vi "短信通知-发送.vi"(11 "探头名称":string) -> ()   [LabVIEW 2017]
uses:
  <vilib>/httpClient/LabVIEWHTTPClient.lvlib
panel:
  out "headers":string caption="头部"
  out "body":string caption="体部"
  out "短信内容":string
  out "Result":string caption="结果"
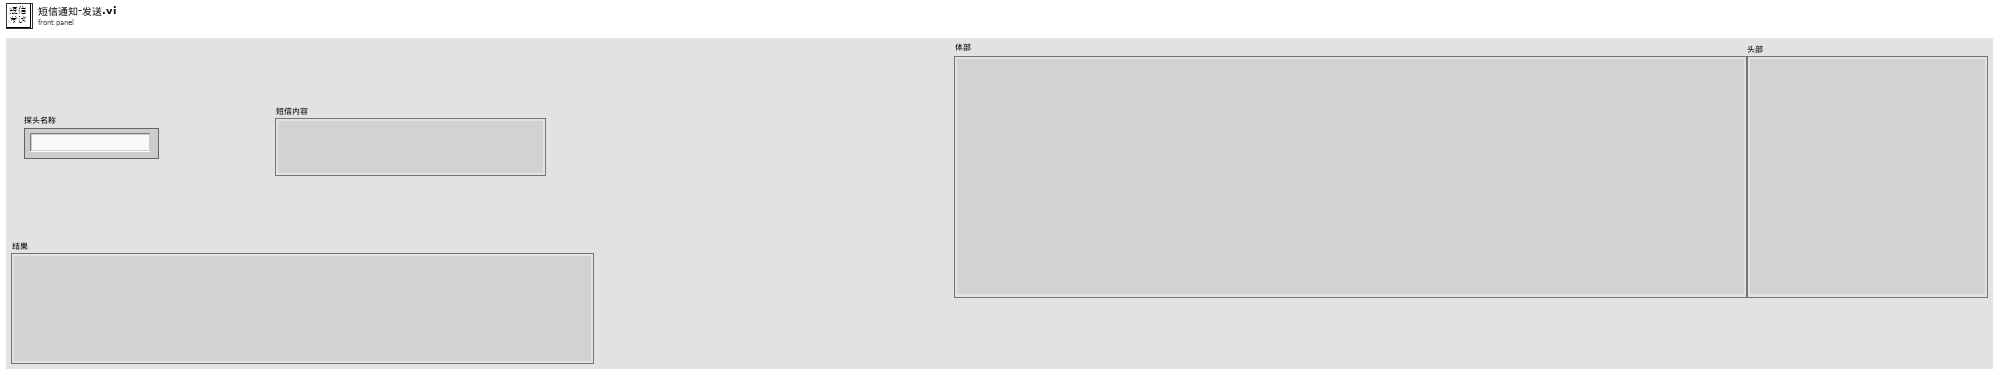
[diagram p1: front panel]
types:
  T1 = cluster{"企业编号":string, "员工编号":string, "通道号":string, "密码":string, "联系人数组":cluster{"姓名":string, "手机号":string}[]}
  T2 = typedef "LabVIEWHTTPClient.lvlib/ClientHandle.ctl" = refnum<k1>
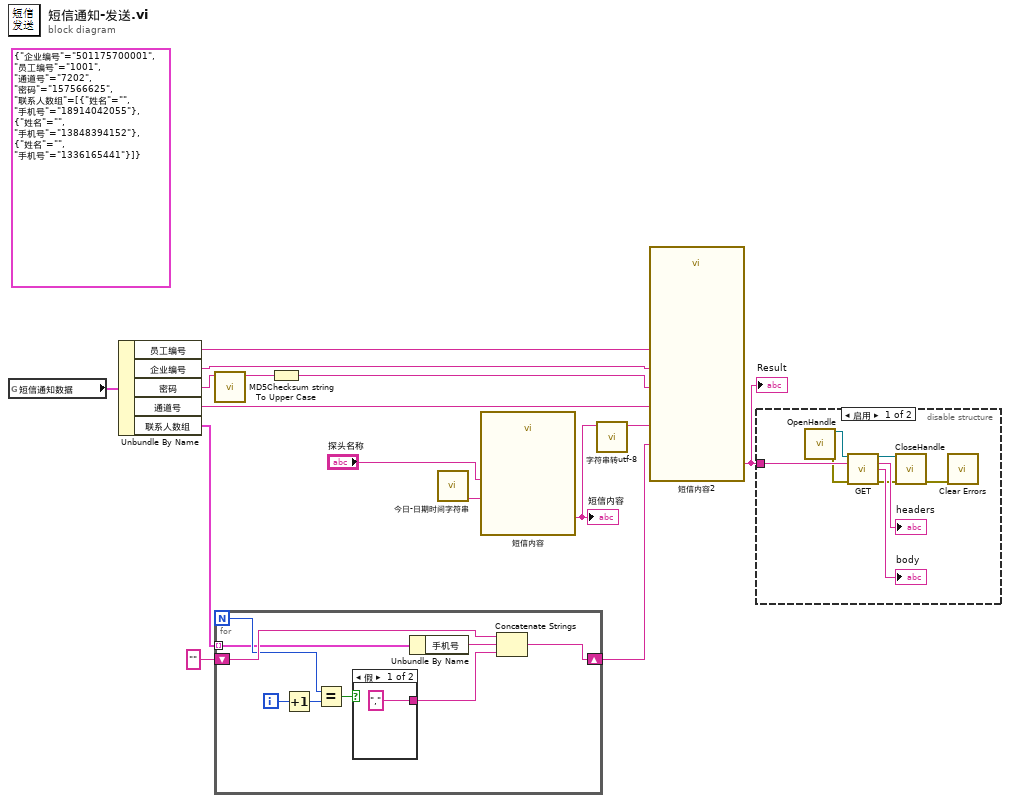
[diagram p0: block diagram]
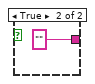
[diagram p3: hidden frame]
diagram:
  (unwired) T1 {"企业编号"="501175700001", "员工编号"="1001", "通道号"="7202", "密码"="157566625", "联系人数组"=[{"姓名"="", "手机号"="18914042055"}, {"姓名"="", "手机号"="13848394152"}, {"姓名"="", "手机号"="1336165441"}]} ("短信通知数据")
  n1 = global read "全局变量-35点监测.vi" "短信通知数据"() -> (w1:T1)
  n2 = Unbundle By Name(w1) -> ("员工编号"=w15:string, "企业编号"=w14:string, "密码"=w12:string, "通道号"=w13:string, "联系人数组"=w9:cluster{"姓名":string, "手机号":string}[])
  n3 = call <vilib>:"MD5Checksum string.vi"("Message String"=w12) -> ("MD5 message-digest"=w11:string)  [unwired: 10 in]
  n4 = for {
    N -> [w19]
    tunnel: w9 -> [w17] mode=indexing
    shift-right: [w23] -> w7
    shift-left: "" -> [w24]
    i -> [w21]
    n5 = Increment(x=w21) -> (x+1=w20:i32)
    n6 = Equal?(x=w19, y=w20) -> (x = y?=w18:bool)
    n7 = case shown="假" w18 {
      tunnel: ["," ("字符串") "" ("字符串")] -> w22
      frame False {
      }
      frame True {
      }
    }
    n8 = Unbundle By Name(w17) -> ("手机号"=w16:string)
    n9 = Concatenate Strings(w24, w16, w22) -> (w23:string)
  }
  n10 = To Upper Case(1:w11) -> (0:w10:string)
  n11 = call "今日-日期时间字符串.vi"() -> ("日期时间"=w4:string)  [unwired: 9 in, 2 out]
  n12 = call "短信内容"("探头名称"="探头名称", "时间"=w4) -> ("Result"=w3:string)  [unwired: 12 in, 1 out]
  "短信内容" <- w3
  n13 = call "字符串转utf-8.vi"("文本"=w3) -> ("utf-8文本"=w6:string)  [unwired: 9 in, 1 out]
  n14 = call "短信内容2"("通道号"=w13, "手机号s"=w7, "员工编号"=w15, "企业编号"=w14, "MD5密码"=w10, "短信内容"=w6) -> ("Result"=w2:string)  [unwired: 8 in, 1 out]
  "Result" <- w2
  n15 = disable-structure shown="启用" {
    disable-tunnel: w2 -> [w31 _]
    frame Enabled {
      n16 = call <vilib>:"OpenHandle.vi"() -> ("client handle out"=w30:T2, "error out"=w29:errorcluster)  [unwired: 14 in]
      n17 = call <vilib>:"GET.vi"("client handle"=w30, "url"=w31, "error in (no error)"=w29) -> ("client handle out"=w32:T2, "headers"=→"headers":string, "body"=→"body":string, "error out"=w28:errorcluster)  [unwired: 9 in]
      n18 = call <vilib>:"CloseHandle.vi"("client handle"=w32, "error in (no error)"=w28) -> ("error out"=w27:errorcluster)  [unwired: 13 in]
      n19 = call <vilib>:"Clear Errors.vi"("error in (no error)"=w27) -> ()  [unwired: 5 in, 2 out]
    }
    frame Disabled {
    }
  }
